vi "MTMount_putSample_AuxiliaryBoxes.vi"(8 "error in (no error)":errorcluster, 11 "Auxiliary_Boxes_Ctl":T1) -> (0 "error out":errorcluster, 2 "function return":i32, 3 "Auxiliary_Boxes_Ctl out":T1)   [LabVIEW 2018, in "SALLV_MTMount.lvlib"]
doc: "int MTMount_shm_putSample_Auxiliary_BoxesLV(MTMount_Auxiliary_BoxesLV *Auxiliary_Boxes_Ctl );"
uses:
  SALLV_MTMount.lvlib
  DataTypes/Auxiliary_Boxes.ctl
  SALLV_MTMount.so
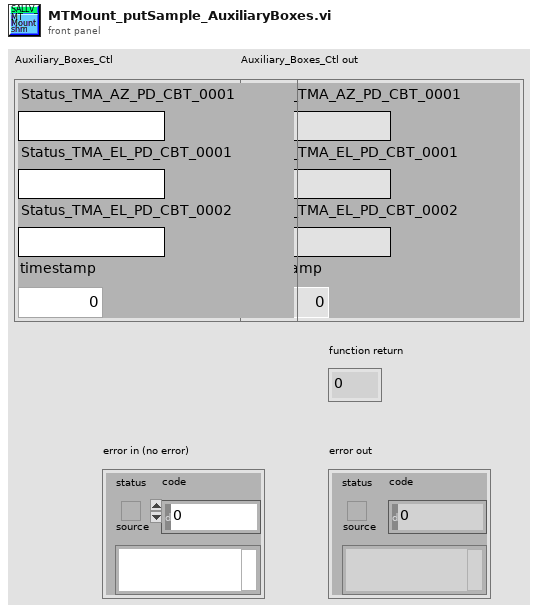
[diagram p1: front panel]
types:
  T1 = typedef "SALLV_MTMount.lvlib/Auxiliary_Boxes.ctl" = cluster{"Status_TMA_AZ_PD_CBT_0001":string, "Status_TMA_EL_PD_CBT_0001":string, "Status_TMA_EL_PD_CBT_0002":string, "timestamp":dbl}
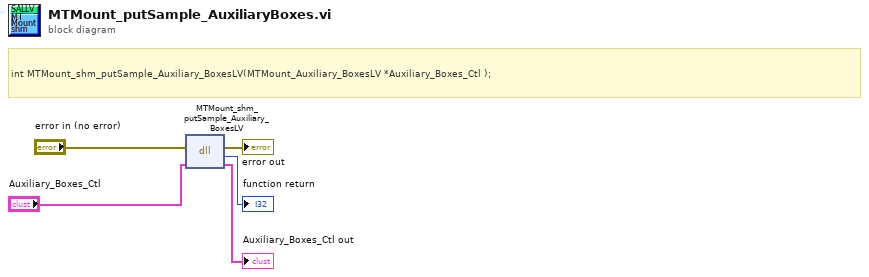
[diagram p0: block diagram]
diagram:
  # "int MTMount_shm_putSample_Auxiliary_BoxesLV(MTMount_Auxiliary_BoxesLV *Auxiliary_Boxes_Ctl );"
  n1 = dll-call lib="home/ttsai/Document/salApiMTMount/SALLV_MTMount/SALLV_MTMount.*" fn="MTMount_shm_putSample_Auxiliary_BoxesLV"(error in="error in (no error)", "Auxiliary_Boxes_Ctl"="Auxiliary_Boxes_Ctl") -> (error out=→"error out":errorcluster, →"function return":i32, "Auxiliary_Boxes_Ctl"=→"Auxiliary_Boxes_Ctl out":T1)  [unwired: 2 in, 1 out]
